vi "FaulhaberV3-Ascii_V1.vi"() -> (1 "searchnames":string[](array[string]), 2 "ID":u32[](array[numeric]), 3 "Faulhaber Objects":T3(array[cluster]))   [LabVIEW 2011] (continued)
Omapping=\"no\" objFlags=\"00020003\" />\n\t\t\t\t\t\t<CANopenSubObject subIndex=\"02\" name=\"Call stack level 1\" objectType=\"7\" dataType=\"0006\" accessType=\"ro\" defaultValue=\"0x0\" PDOmapping=\"no\" objFlags=\"00020003\" />\n\t\t\t\t\t\t<CANopenSubObject subIndex=\"03\" name=\"Call stack level 2\" objectType=\"7\" dataType=\"0006\" accessType=\"ro\" defaultValue=\"0x0\" PDOmapping=\"no\" objFlags=\"00020003\" />\n\t\t\t\t\t\t<CANopenSubObject subIndex=\"04\" name=\"Call stack level 3\" objectType=\"7\" dataType=\"0006\" accessType=\"ro\" defaultValue=\"0x0\" PDOmapping=\"no\" objFlags=\"00020003\" />\n\t\t\t\t\t\t<CANopenSubObject subIndex=\"05\" name=\"Call stack level 4\" objectType=\"7\" dataType=\"0006\" accessType=\"ro\" defaultValue=\"0x0\" PDOmapping=\"no\" objFlags=\"00020003\" />\n\t\t\t\t\t\t<CANopenSubObject subIndex=\"06\" name=\"Call stack level 5\" objectType=\"7\" dataType=\"0006\" accessType=\"ro\" defaultValue=\"0x0\" PDOmapping=\"no\" objFlags=\"00020003\" />\n\t\t\t\t\t\t<CANopenSubObject subIndex=\"07\" name=\"Call stack level 6\" objectType=\"7\" dataType=\"0006\" accessType=\"ro\" defaultValue=\"0x0\" PDOmapping=\"no\" objFlags=\"00020003\" />\n\t\t\t\t\t\t<CANopenSubObject subIndex=\"08\" name=\"Call stack level 7\" objectType=\"7\" dataType=\"0006\" accessType=\"ro\" defaultValue=\"0x0\" PDOmapping=\"no\" objFlags=\"00020003\" />\n\t\t\t\t\t\t<CANopenSubObject subIndex=\"09\" name=\"Call stack level 8\" objectType=\"7\" dataType=\"0006\" accessType=\"ro\" defaultValue=\"0x0\" PDOmapping=\"no\" objFlags=\"00020003\" />\n\t\t\t\t\t\t<CANopenSubObject subIndex=\"0A\" name=\"Call stack level 9\" objectType=\"7\" dataType=\"0006\" accessType=\"ro\" defaultValue=\"0x0\" PDOmapping=\"no\" objFlags=\"00020003\" />\n\t\t\t\t\t\t<CANopenSubObject subIndex=\"0B\" name=\"Call stack level 10\" objectType=\"7\" dataType=\"0006\" accessType=\"ro\" defaultValue=\"0x0\" PDOmapping=\"no\" objFlags=\"00020003\" />\n\t\t\t\t\t\t<CANopenSubObject subIndex=\"0C\" name=\"Call stack level 11\" objectType=\"7\" dataType=\"0006\" accessType=\"ro\" defaultValue=\"0x0\" PDOmapping=\"no\" objFlags=\"00020003\" />\n\t\t\t\t\t\t<CANopenSubObject subIndex=\"0D\" name=\"Call stack level 12\" objectType=\"7\" dataType=\"0006\" accessType=\"ro\" defaultValue=\"0x0\" PDOmapping=\"no\" objFlags=\"00020003\" />\n\t\t\t\t\t\t<CANopenSubObject subIndex=\"0E\" name=\"Call stack level 13\" objectType=\"7\" dataType=\"0006\" accessType=\"ro\" defaultValue=\"0x0\" PDOmapping=\"no\" objFlags=\"00020003\" />\n\t\t\t\t\t\t<CANopenSubObject subIndex=\"0F\" name=\"Call stack level 14\" objectType=\"7\" dataType=\"0006\" accessType=\"ro\" defaultValue=\"0x0\" PDOmapping=\"no\" objFlags=\"00020003\" />\n\t\t\t\t\t</CANopenObject>\n\t\t\t\t\t<CANopenObject index=\"300F\" name=\"Variable access key\" objectType=\"7\" dataType=\"0007\" lowLimit=\"0\" highLimit=\"4294967295\" accessType=\"wo\" defaultValue=\"0\" PDOmapping=\"TPDO\" objFlags=\"00020000\" />\n\t\t\t\t\t<CANopenObject index=\"3010\" name=\"Program constants\" objectType=\"9\" subNumber=\"17\">\n\t\t\t\t\t\t<CANopenSubObject subIndex=\"00\" name=\"Number of entries\" objectType=\"7\" dataType=\"0005\" accessType=\"ro\" defaultValue=\"16\" PDOmapping=\"no\" />\n\t\t\t\t\t\t<CANopenSubObject subIndex=\"01\" name=\"Program constant 0\" objectType=\"7\" dataType=\"0004\" lowLimit=\"-2147483648\" highLimit=\"2147483647\" accessType=\"rw\" defaultValue=\"0\" PDOmapping=\"optional\" />\n\t\t\t\t\t\t<CANopenSubObject subIndex=\"02\" name=\"Program constant 1\" objectType=\"7\" dataType=\"0004\" lowLimit=\"-2147483648\" highLimit=\"2147483647\" accessType=\"rw\" defaultValue=\"0\" PDOmapping=\"optional\" />\n\t\t\t\t\t\t<CANopenSubObject subIndex=\"03\" name=\"Program constant 2\" objectType=\"7\" dataType=\"0004\" lowLimit=\"-2147483648\" highLimit=\"2147483647\" accessType=\"rw\" defaultValue=\"0\" PDOmapping=\"optional\" />\n\t\t\t\t\t\t<CANopenSubObject subIndex=\"04\" name=\"Program constant 3\" objectType=\"7\" dataType=\"0004\" lowLimit=\"-2147483648\" highLimit=\"2147483647\" accessType=\"rw\" defaultValue=\"0\" PDOmapping=\"optional\" />\n\t\t\t\t\t\t<CANopenSubObject subIndex=\"05\" name=\"Program constant 4\" objectType=\"7\" dataType=\"0004\" lowLimit=\"-2147483648\" highLimit=\"2147483647\" accessType=\"rw\" defaultValue=\"0\" PDOmapping=\"optional\" />\n\t\t\t\t\t\t<CANopenSubObject subIndex=\"06\" name=\"Program constant 5\" objectType=\"7\" dataType=\"0004\" lowLimit=\"-2147483648\" highLimit=\"2147483647\" accessType=\"rw\" defaultValue=\"0\" PDOmapping=\"optional\" />\n\t\t\t\t\t\t<CANopenSubObject subIndex=\"07\" name=\"Program constant 6\" objectType=\"7\" dataType=\"0004\" lowLimit=\"-2147483648\" highLimit=\"2147483647\" accessType=\"rw\" defaultValue=\"0\" PDOmapping=\"optional\" />\n\t\t\t\t\t\t<CANopenSubObject subIndex=\"08\" name=\"Program constant 7\" objectType=\"7\" dataType=\"0004\" lowLimit=\"-2147483648\" highLimit=\"2147483647\" accessType=\"rw\" defaultValue=\"0\" PDOmapping=\"optional\" />\n\t\t\t\t\t\t<CANopenSubObject subIndex=\"09\" name=\"Program constant 8\" objectType=\"7\" dataType=\"0004\" lowLimit=\"-2147483648\" highLimit=\"2147483647\" accessType=\"rw\" defaultValue=\"0\" PDOmapping=\"optional\" />\n\t\t\t\t\t\t<CANopenSubObject subIndex=\"0A\" name=\"Program constant 9\" objectType=\"7\" dataType=\"0004\" lowLimit=\"-2147483648\" highLimit=\"2147483647\" accessType=\"rw\" defaultValue=\"0\" PDOmapping=\"optional\" />\n\t\t\t\t\t\t<CANopenSubObject subIndex=\"0B\" name=\"Program constant 10\" objectType=\"7\" dataType=\"0004\" lowLimit=\"-2147483648\" highLimit=\"2147483647\" accessType=\"rw\" defaultValue=\"0\" PDOmapping=\"optional\" />\n\t\t\t\t\t\t<CANopenSubObject subIndex=\"0C\" name=\"Program constant 11\" objectType=\"7\" dataType=\"0004\" lowLimit=\"-2147483648\" highLimit=\"2147483647\" accessType=\"rw\" defaultValue=\"0\" PDOmapping=\"optional\" />\n\t\t\t\t\t\t<CANopenSubObject subIndex=\"0D\" name=\"Program constant 12\" objectType=\"7\" dataType=\"0004\" lowLimit=\"-2147483648\" highLimit=\"2147483647\" accessType=\"rw\" defaultValue=\"0\" PDOmapping=\"optional\" />\n\t\t\t\t\t\t<CANopenSubObject subIndex=\"0E\" name=\"Program constant 13\" objectType=\"7\" dataType=\"0004\" lowLimit=\"-2147483648\" highLimit=\"2147483647\" accessType=\"rw\" defaultValue=\"0\" PDOmapping=\"optional\" />\n\t\t\t\t\t\t<CANopenSubObject subIndex=\"0F\" name=\"Program constant 14\" objectType=\"7\" dataType=\"0004\" lowLimit=\"-2147483648\" highLimit=\"2147483647\" accessType=\"rw\" defaultValue=\"0\" PDOmapping=\"optional\" />\n\t\t\t\t\t\t<CANopenSubObject subIndex=\"10\" name=\"Program constant 15\" objectType=\"7\" dataType=\"0004\" lowLimit=\"-2147483648\" highLimit=\"2147483647\" accessType=\"rw\" defaultValue=\"0\" PDOmapping=\"optional\" />\n\t\t\t\t\t</CANopenObject>\n\t\t\t\t\t<CANopenObject index=\"6007\" name=\"Abort connection option code\" objectType=\"7\" dataType=\"0003\" PDOmapping=\"RPDO\" objFlags=\"00020000\" uniqueIDRef=\"UID_PARAM_6007\" />\n\t\t\t\t\t<CANopenObject index=\"6040\" name=\"Controlword\" objectType=\"7\" dataType=\"0006\" lowLimit=\"0\" highLimit=\"65535\" accessType=\"rw\" defaultValue=\"0x0\" PDOmapping=\"RPDO\" objFlags=\"0001\" />\n\t\t\t\t\t<CANopenObject index=\"6041\" name=\"Statusword\" objectType=\"7\" dataType=\"0006\" lowLimit=\"0x0\" accessType=\"ro\" PDOmapping=\"TPDO\" />\n\t\t\t\t\t<CANopenObject index=\"605A\" name=\"Quick-Stop option code\" objectType=\"7\" dataType=\"0003\" PDOmapping=\"RPDO\" objFlags=\"00020000\" uniqueIDRef=\"UID_PARAM_605A\" />\n\t\t\t\t\t<CANopenObject index=\"605B\" name=\"Shutdown option code\" objectType=\"7\" dataType=\"0003\" PDOmapping=\"RPDO\" objFlags=\"00020000\" uniqueIDRef=\"UID_PARAM_605B\" />\n\t\t\t\t\t<CANopenObject index=\"605C\" name=\"Disable operation option code\" objectType=\"7\" dataType=\"0003\" PDOmapping=\"RPDO\" objFlags=\"00020000\" uniqueIDRef=\"UID_PARAM_605C\" />\n\t\t\t\t\t<CANopenObject index=\"605D\" name=\"Halt option code\" objectType=\"7\" dataType=\"0003\" PDOmapping=\"RPDO\" objFlags=\"00020000\" uniqueIDRef=\"UID_PARAM_605D\" />\n\t\t\t\t\t<CANopenObject index=\"605E\" name=\"Fault reaction option code\" objectType=\"7\" dataType=\"0003\" PDOmapping=\"RPDO\" objFlags=\"00020000\" uniqueIDRef=\"UID_PARAM_605E\" />\n\t\t\t\t\t<CANopenObject index=\"6060\" name=\"Modes of operation\" objectType=\"7\" dataType=\"0002\" PDOmapping=\"RPDO\" objFlags=\"00020000\" uniqueIDRef=\"UID_PARAM_6060\" />\n\t\t\t\t\t<CANopenObject index=\"6061\" name=\"Modes of operation display\" objectType=\"7\" dataType=\"0002\" accessType=\"ro\" PDOmapping=\"TPDO\" objFlags=\"00020000\" />\n\t\t\t\t\t<CANopenObject index=\"6062\" name=\"Position demand value\" objectType=\"7\" dataType=\"0004\" accessType=\"ro\" PDOmapping=\"TPDO\" />\n\t\t\t\t\t<CANopenObject index=\"6063\" name=\"Position actual internal value\" objectType=\"7\" dataType=\"0004\" accessType=\"ro\" PDOmapping=\"TPDO\" />\n\t\t\t\t\t<CANopenObject index=\"6064\" name=\"Position actual value\" objectType=\"7\" dataType=\"0004\" accessType=\"ro\" PDOmapping=\"TPDO\" />\n\t\t\t\t\t<CANopenObject index=\"6065\" name=\"Following error window\" objectType=\"7\" dataType=\"0007\" lowLimit=\"0\" highLimit=\"4294967295\" accessType=\"rw\" PDOmapping=\"RPDO\" objFlags=\"00020000\" />\n\t\t\t\t\t<CANopenObject index=\"6066\" name=\"Following error time out\" objectType=\"7\" dataType=\"0006\" lowLimit=\"1\" highLimit=\"65535\" accessType=\"rw\" PDOmapping=\"RPDO\" objFlags=\"00020000\" />\n\t\t\t\t\t<CANopenObject index=\"6067\" name=\"Position window\" objectType=\"7\" dataType=\"0007\" lowLimit=\"0\" highLimit=\"4294967295\" accessType=\"rw\" PDOmapping=\"RPDO\" objFlags=\"00020000\" />\n\t\t\t\t\t<CANopenObject index=\"6068\" name=\"Position window time\" objectType=\"7\" dataType=\"0006\" lowLimit=\"1\" highLimit=\"65535\" accessType=\"rw\" PDOmapping=\"RPDO\" objFlags=\"00020000\" />\n\t\t\t\t\t<CANopenObject index=\"606B\" name=\"Velocity demand value\" objectType=\"7\" dataType=\"0004\" accessType=\"ro\" PDOmapping=\"TPDO\" />\n\t\t\t\t\t<CANopenObject index=\"606C\" name=\"Velocity actual value\" objectType=\"7\" dataType=\"0004\" accessType=\"ro\" PDOmapping=\"TPDO\" />\n\t\t\t\t\t<CANopenObject index=\"606D\" name=\"Velocity window\" objectType=\"7\" dataType=\"0006\" lowLimit=\"0\" highLimit=\"65535\" accessType=\"rw\" PDOmapping=\"RPDO\" objFlags=\"00020000\" />\n\t\t\t\t\t<CANopenObject index=\"606E\" name=\"Velocity window time\" objectType=\"7\" dataType=\"0006\" lowLimit=\"1\" highLimit=\"65535\" accessType=\"rw\" PDOmapping=\"RPDO\" objFlags=\"00020000\" />\n\t\t\t\t\t<CANopenObject index=\"606F\" name=\"Velocity threshold\" objectType=\"7\" dataType=\"0006\" lowLimit=\"0\" highLimit=\"65535\" accessType=\"rw\" PDOmapping=\"RPDO\" objFlags=\"00020000\" />\n\t\t\t\t\t<CANopenObject index=\"6070\" name=\"Velocity threshold time\" objectType=\"7\" dataType=\"0006\" lowLimit=\"1\" highLimit=\"65535\" accessType=\"rw\" PDOmapping=\"RPDO\" objFlags=\"00020000\" />\n\t\t\t\t\t<CANopenObject index=\"6071\" name=\"Target torque\" objectType=\"7\" dataType=\"0003\" lowLimit=\"-32768\" highLimit=\"32767\" accessType=\"rw\" defaultValue=\"0\" PDOmapping=\"RPDO\" />\n\t\t\t\t\t<CANopenObject index=\"6072\" name=\"Max torque\" objectType=\"7\" dataType=\"0006\" accessType=\"ro\" PDOmapping=\"TPDO\" />\n\t\t\t\t\t<CANopenObject index=\"6074\" name=\"Torque demand\" objectType=\"7\" dataType=\"0003\" accessType=\"ro\" PDOmapping=\"TPDO\" />\n\t\t\t\t\t<CANopenObject index=\"6077\" name=\"Torque actual value\" objectType=\"7\" dataType=\"0003\" accessType=\"ro\" PDOmapping=\"TPDO\" />\n\t\t\t\t\t<CANopenObject index=\"6078\" name=\"Current actual value\" objectType=\"7\" dataType=\"0003\" accessType=\"ro\" PDOmapping=\"TPDO\" />\n\t\t\t\t\t<CANopenObject index=\"607A\" name=\"Target position\" objectType=\"7\" dataType=\"0004\" lowLimit=\"-2147483648\" highLimit=\"2147483647\" accessType=\"rw\" defaultValue=\"0\" PDOmapping=\"RPDO\" />\n\t\t\t\t\t<CANopenObject index=\"607B\" name=\"Position range limit\" objectType=\"8\" subNumber=\"3\">\n\t\t\t\t\t\t<CANopenSubObject subIndex=\"00\" name=\"Number of entries\" objectType=\"7\" dataType=\"0005\" accessType=\"ro\" defaultValue=\"2\" PDOmapping=\"no\" />\n\t\t\t\t\t\t<CANopenSubObject subIndex=\"01\" name=\"Min position range limit\" objectType=\"7\" dataType=\"0004\" lowLimit=\"-2147483648\" highLimit=\"2147483647\" accessType=\"rw\" defaultValue=\"-2147483648\" PDOmapping=\"RPDO\" objFlags=\"00020000\" />\n\t\t\t\t\t\t<CANopenSubObject subIndex=\"02\" name=\"Max position range limit\" objectType=\"7\" dataType=\"0004\" lowLimit=\"-2147483648\" highLimit=\"2147483647\" accessType=\"rw\" defaultValue=\"2147483647\" PDOmapping=\"RPDO\" objFlags=\"00020000\" />\n\t\t\t\t\t</CANopenObject>\n\t\t\t\t\t<CANopenObject index=\"607C\" name=\"Home offset\" objectType=\"7\" dataType=\"0004\" lowLimit=\"-2147483648\" highLimit=\"2147483647\" accessType=\"rw\" defaultValue=\"0\" PDOmapping=\"RPDO\" objFlags=\"00020000\" />\n\t\t\t\t\t<CANopenObject index=\"607D\" name=\"Software position limit\" objectType=\"8\" subNumber=\"3\">\n\t\t\t\t\t\t<CANopenSubObject subIndex=\"00\" name=\"Number of entries\" objectType=\"7\" dataType=\"0005\" accessType=\"ro\" defaultValue=\"2\" PDOmapping=\"no\" />\n\t\t\t\t\t\t<CANopenSubObject subIndex=\"01\" name=\"Min position limit\" objectType=\"7\" dataType=\"0004\" lowLimit=\"-2147483648\" highLimit=\"2147483647\" accessType=\"rw\" defaultValue=\"-2147483648\" PDOmapping=\"RPDO\" objFlags=\"00020000\" />\n\t\t\t\t\t\t<CANopenSubObject subIndex=\"02\" name=\"Max position limit\" objectType=\"7\" dataType=\"0004\" lowLimit=\"-2147483648\" highLimit=\"2147483647\" accessType=\"rw\" defaultValue=\"2147483647\" PDOmapping=\"RPDO\" objFlags=\"00020000\" />\n\t\t\t\t\t</CANopenObject>\n\t\t\t\t\t<CANopenObject index=\"607E\" name=\"Polarity\" objectType=\"7\" dataType=\"0005\" PDOmapping=\"RPDO\" objFlags=\"00020000\" uniqueIDRef=\"UID_PARAM_607E\" />\n\t\t\t\t\t<CANopenObject index=\"6080\" name=\"Max motor speed \" objectType=\"7\" dataType=\"0007\" lowLimit=\"1\" highLimit=\"4294967295\" accessType=\"rw\" defaultValue=\"32767\" PDOmapping=\"RPDO\" />\n\t\t\t\t\t<CANopenObject index=\"6081\" name=\"Profile velocity\" objectType=\"7\" dataType=\"0007\" lowLimit=\"1\" highLimit=\"4294967295\" accessType=\"rw\" defaultValue=\"32767\" PDOmapping=\"RPDO\" />\n\t\t\t\t\t<CANopenObject index=\"6083\" name=\"Profile acceleration\" objectType=\"7\" dataType=\"0007\" lowLimit=\"1\" highLimit=\"32767\" accessType=\"rw\" defaultValue=\"30000\" PDOmapping=\"RPDO\" />\n\t\t\t\t\t<CANopenObject index=\"6084\" name=\"Profile deceleration\" objectType=\"7\" dataType=\"0007\" lowLimit=\"1\" highLimit=\"32767\" accessType=\"rw\" defaultValue=\"30000\" PDOmapping=\"RPDO\" />\n\t\t\t\t\t<CANopenObject index=\"6085\" name=\"Quick stop deceleration\" objectType=\"7\" dataType=\"0007\" lowLimit=\"10\" highLimit=\"32767\" accessType=\"rw\" defaultValue=\"30000\" PDOmapping=\"RPDO\" />\n\t\t\t\t\t<CANopenObject index=\"6086\" name=\"Motion profile type\" objectType=\"7\" dataType=\"0003\" PDOmapping=\"RPDO\" objFlags=\"00020000\" uniqueIDRef=\"UID_PARAM_6086\" />\n\t\t\t\t\t<CANopenObject index=\"608F\" name=\"Position encoder resolution\" objectType=\"8\" subNumber=\"3\">\n\t\t\t\t\t\t<CANopenSubObject subIndex=\"00\" name=\"Number of entries\" objectType=\"7\" dataType=\"0005\" accessType=\"ro\" defaultValue=\"2\" PDOmapping=\"no\" />\n\t\t\t\t\t\t<CANopenSubObject subIndex=\"01\" name=\"Encoder increments\" objectType=\"7\" dataType=\"0007\" accessType=\"ro\" PDOmapping=\"no\" objFlags=\"00020000\" />\n\t\t\t\t\t\t<CANopenSubObject subIndex=\"02\" name=\"Motor revolutions\" objectType=\"7\" dataType=\"0007\" accessType=\"ro\" PDOmapping=\"no\" objFlags=\"00020000\" />\n\t\t\t\t\t</CANopenObject>\n\t\t\t\t\t<CANopenObject index=\"6090\" name=\"Velocity encoder resolution\" objectType=\"8\" subNumber=\"3\">\n\t\t\t\t\t\t<CANopenSubObject subIndex=\"00\" name=\"Number of entries\" objectType=\"7\" dataType=\"0005\" accessType=\"ro\" defaultValue=\"2\" PDOmapping=\"no\" />\n\t\t\t\t\t\t<CANopenSubObject subIndex=\"01\" name=\"Encoder increments\" objectType=\"7\" dataType=\"0007\" accessType=\"ro\" PDOmapping=\"no\" objFlags=\"00020000\" />\n\t\t\t\t\t\t<CANopenSubObject subIndex=\"02\" name=\"Motor revolutions\" objectType=\"7\" dataType=\"0007\" accessType=\"ro\" PDOmapping=\"no\" objFlags=\"00020000\" />\n\t\t\t\t\t</CANopenObject>\n\t\t\t\t\t<CANopenObject index=\"6091\" name=\"Gear ratio\" objectType=\"8\" subNumber=\"3\">\n\t\t\t\t\t\t<CANopenSubObject subIndex=\"00\" name=\"Number of entries\" objectType=\"7\" dataType=\"0005\" accessType=\"ro\" defaultValue=\"2\" PDOmapping=\"no\" />\n\t\t\t\t\t\t<CANopenSubObject subIndex=\"01\" name=\"Motor shaft revolutions\" objectType=\"7\" dataType=\"0007\" lowLimit=\"1\" highLimit=\"4294967295\" accessType=\"rw\" defaultValue=\"1\" PDOmapping=\"RPDO\" objFlags=\"00020000\" />\n\t\t\t\t\t\t<CANopenSubObject subIndex=\"02\" name=\"Driving shaft revolutions\" objectType=\"7\" dataType=\"0007\" lowLimit=\"1\" highLimit=\"4294967295\" accessType=\"rw\" defaultValue=\"1\" PDOmapping=\"RPDO\" objFlags=\"00020000\" />\n\t\t\t\t\t</CANopenObject>\n\t\t\t\t\t<CANopenObject index=\"6092\" name=\"Feed constant\" objectType=\"8\" subNumber=\"3\">\n\t\t\t\t\t\t<CANopenSubObject subIndex=\"00\" name=\"Number of entries\" objectType=\"7\" dataType=\"0005\" accessType=\"ro\" defaultValue=\"2\" PDOmapping=\"no\" />\n\t\t\t\t\t\t<CANopenSubObject subIndex=\"01\" name=\"Feed\" objectType=\"7\" dataType=\"0007\" lowLimit=\"1\" highLimit=\"4294967295\" accessType=\"rw\" defaultValue=\"4096\" PDOmapping=\"RPDO\" objFlags=\"00020000\" />\n\t\t\t\t\t\t<CANopenSubObject subIndex=\"02\" name=\"Shaft revolutions\" objectType=\"7\" dataType=\"0007\" lowLimit=\"1\" highLimit=\"4294967295\" accessType=\"rw\" defaultValue=\"1\" PDOmapping=\"RPDO\" objFlags=\"00020000\" />\n\t\t\t\t\t</CANopenObject>\n\t\t\t\t\t<CANopenObject index=\"6096\" name=\"Velocity factor\" objectType=\"8\" subNumber=\"3\">\n\t\t\t\t\t\t<CANopenSubObject subIndex=\"00\" name=\"Number of entries\" objectType=\"7\" dataType=\"0005\" accessType=\"ro\" defaultValue=\"2\" PDOmapping=\"no\" />\n\t\t\t\t\t\t<CANopenSubObject subIndex=\"01\" name=\"Numerator\" objectType=\"7\" dataType=\"0007\" lowLimit=\"1\" highLimit=\"4294967295\" accessType=\"rw\" defaultValue=\"1\" PDOmapping=\"RPDO\" objFlags=\"00020000\" />\n\t\t\t\t\t\t<CANopenSubObject subIndex=\"02\" name=\"Divisor\" objectType=\"7\" dataType=\"0007\" lowLimit=\"1\" highLimit=\"4294967295\" accessType=\"rw\" defaultValue=\"4096\" PDOmapping=\"RPDO\" objFlags=\"00020000\" />\n\t\t\t\t\t</CANopenObject>\n\t\t\t\t\t<CANopenObject index=\"6098\" name=\"Homing method\" objectType=\"7\" dataType=\"0002\" lowLimit=\"-4\" highLimit=\"37\" accessType=\"rw\" defaultValue=\"0\" PDOmapping=\"RPDO\" objFlags=\"00020000\" />\n\t\t\t\t\t<CANopenObject index=\"6099\" name=\"Homing speeds\" objectType=\"8\" subNumber=\"3\">\n\t\t\t\t\t\t<CANopenSubObject subIndex=\"00\" name=\"Number of entries\" objectType=\"7\" dataType=\"0005\" accessType=\"ro\" defaultValue=\"2\" PDOmapping=\"no\" />\n\t\t\t\t\t\t<CANopenSubObject subIndex=\"01\" name=\"Switch seek velocity\" objectType=\"7\" dataType=\"0007\" lowLimit=\"0\" highLimit=\"4294967295\" accessType=\"rw\" defaultValue=\"400\" PDOmapping=\"RPDO\" objFlags=\"00020000\" />\n\t\t\t\t\t\t<CANopenSubObject subIndex=\"02\" name=\"Homing speed\" objectType=\"7\" dataType=\"0007\" lowLimit=\"0\" highLimit=\"4294967295\" accessType=\"rw\" defaultValue=\"400\" PDOmapping=\"RPDO\" objFlags=\"00020000\" />\n\t\t\t\t\t</CANopenObject>\n\t\t\t\t\t<CANopenObject index=\"609A\" name=\"Homing acceleration\" objectType=\"7\" dataType=\"0007\" lowLimit=\"0\" highLimit=\"4294967295\" accessType=\"rw\" defaultValue=\"50\" PDOmapping=\"RPDO\" objFlags=\"00020000\" />\n\t\t\t\t\t<CANopenObject index=\"60B0\" name=\"Position offset\" objectType=\"7\" dataType=\"0004\" lowLimit=\"-2147483648\" highLimit=\"2147483647\" accessType=\"rw\" defaultValue=\"0\" PDOmapping=\"RPDO\" />\n\t\t\t\t\t<CANopenObject index=\"60B1\" name=\"Velocity offset\" objectType=\"7\" dataType=\"0004\" lowLimit=\"-2147483648\" highLimit=\"2147483647\" accessType=\"rw\" defaultValue=\"0\" PDOmapping=\"RPDO\" />\n\t\t\t\t\t<CANopenObject index=\"60B2\" name=\"Torque offset\" objectType=\"7\" dataType=\"0003\" lowLimit=\"-32768\" highLimit=\"32767\" accessType=\"rw\" defaultValue=\"0\" PDOmapping=\"RPDO\" />\n\t\t\t\t\t<CANopenObject index=\"60B8\" name=\"Touch probe function\" objectType=\"7\" dataType=\"0006\" accessType=\"rw\" defaultValue=\"0\" PDOmapping=\"RPDO\" />\n\t\t\t\t\t<CANopenObject index=\"60B9\" name=\"Touch probe status\" objectType=\"7\" dataType=\"0006\" accessType=\"ro\" defaultValue=\"0x0000\" PDOmapping=\"TPDO\" />\n\t\t\t\t\t<CANopenObject index=\"60BA\" name=\"Touch probe 1 positive edge\" objectType=\"7\" dataType=\"0004\" accessType=\"ro\" defaultValue=\"0x0000\" PDOmapping=\"TPDO\" />\n\t\t\t\t\t<CANopenObject index=\"60BB\" name=\"Touch probe 1 negative edge\" objectType=\"7\" dataType=\"0004\" accessType=\"ro\" PDOmapping=\"TPDO\" />\n\t\t\t\t\t<CANopenObject index=\"60BC\" name=\"Touch probe 2 positive edge\" objectType=\"7\" dataType=\"0004\" accessType=\"ro\" PDOmapping=\"TPDO\" />\n\t\t\t\t\t<CANopenObject index=\"60BD\" name=\"Touch probe 2 negative edge\" objectType=\"7\" dataType=\"0004\" accessType=\"ro\" PDOmapping=\"TPDO\" />\n\t\t\t\t\t<CANopenObject index=\"60C5\" name=\"Max acceleration\" objectType=\"7\" dataType=\"0007\" lowLimit=\"10\" highLimit=\"32767\" accessType=\"rw\" defaultValue=\"30000\" PDOmapping=\"RPDO\" objFlags=\"00020000\" />\n\t\t\t\t\t<CANopenObject index=\"60C6\" name=\"Max deceleration\" objectType=\"7\" dataType=\"0007\" lowLimit=\"10\" highLimit=\"32767\" accessType=\"rw\" defaultValue=\"30000\" PDOmapping=\"RPDO\" objFlags=\"00020000\" />\n\t\t\t\t\t<CANopenObject index=\"60D5\" name=\"Touch probe 1 positive edge counter\" objectType=\"7\" dataType=\"0006\" accessType=\"ro\" PDOmapping=\"TPDO\" />\n\t\t\t\t\t<CANopenObject index=\"60D6\" name=\"Touch probe 1 negative edge counter\" objectType=\"7\" dataType=\"0006\" accessType=\"ro\" PDOmapping=\"TPDO\" />\n\t\t\t\t\t<CANopenObject index=\"60D7\" name=\"Touch probe 2 positive edge counter\" objectType=\"7\" dataType=\"0006\" accessType=\"ro\" PDOmapping=\"TPDO\" />\n\t\t\t\t\t<CANopenObject index=\"60D8\" name=\"Touch probe 2 negative edge counter\" objectType=\"7\" dataType=\"0006\" accessType=\"ro\" PDOmapping=\"TPDO\" />\n\t\t\t\t\t<CANopenObject index=\"60E0\" name=\"Positive torque limit value\" objectType=\"7\" dataType=\"0006\" lowLimit=\"0\" highLimit=\"6000\" accessType=\"rw\" defaultValue=\"2000\" PDOmapping=\"RPDO\" />\n\t\t\t\t\t<CANopenObject index=\"60E1\" name=\"Negative torque limit value\" objectType=\"7\" dataType=\"0006\" lowLimit=\"0\" highLimit=\"6000\" accessType=\"rw\" defaultValue=\"2000\" PDOmapping=\"RPDO\" />\n\t\t\t\t\t<CANopenObject index=\"60F2\" name=\"Position option code\" objectType=\"7\" dataType=\"0006\" PDOmapping=\"RPDO\" objFlags=\"00020000\" uniqueIDRef=\"UID_PARAM_60F2\" />\n\t\t\t\t\t<CANopenObject index=\"60F4\" name=\"Following error actual value\" objectType=\"7\" dataType=\"0004\" accessType=\"ro\" PDOmapping=\"TPDO\" />\n\t\t\t\t\t<CANopenObject index=\"60FD\" name=\"Digital Inputs\" objectType=\"7\" dataType=\"0007\" accessType=\"ro\" PDOmapping=\"TPDO\" />\n\t\t\t\t\t<CANopenObject index=\"60FF\" name=\"Target velocity\" objectType=\"7\" dataType=\"0004\" lowLimit=\"-2147483648\" highLimit=\"2147483647\" accessType=\"rw\" defaultValue=\"0\" PDOmapping=\"RPDO\" />\n\t\t\t\t\t<CANopenObject index=\"6403\" name=\"Motor catalogue number\" objectType=\"7\" dataType=\"0009\" accessType=\"ro\" PDOmapping=\"no\" objFlags=\"00020000\" />\n\t\t\t\t\t<CANopenObject index=\"6502\" name=\"Supported drive modes\" objectType=\"7\" dataType=\"0007\" accessType=\"ro\" PDOmapping=\"TPDO\" objFlags=\"00020000\" />\n\t\t\t\t\t<CANopenObject index=\"6503\" name=\"Drive catalogue number\" objectType=\"7\" dataType=\"0009\" accessType=\"const\" defaultValue=\"0\" PDOmapping=\"no\" objFlags=\"00020000\" />\n\t\t\t\t</CANopenObjectList>\n\t\t\t\t<dummyUsage>\n\t\t\t\t\t<dummy entry=\"Dummy0001=0\" />\n\t\t\t\t\t<dummy entry=\"Dummy0002=0\" />\n\t\t\t\t\t<dummy entry=\"Dummy0003=0\" />\n\t\t\t\t\t<dummy entry=\"Dummy0004=0\" />\n\t\t\t\t\t<dummy entry=\"Dummy0005=0\" />\n\t\t\t\t\t<dummy entry=\"Dummy0006=0\" />\n\t\t\t\t\t<dummy entry=\"Dummy0007=0\" />\n\t\t\t\t</dummyUsage>\n\t\t\t</ApplicationLayers>\n\t\t\t<TransportLayers>\n\t\t\t\t<PhysicalLayer>\n\t\t\t\t\t<baudRate defaultValue=\"250 Kbps\">\n\t\t\t\t\t\t<supportedBaudRate value=\"20 Kbps\" />\n\t\t\t\t\t\t<supportedBaudRate value=\"50 Kbps\" />\n\t\t\t\t\t\t<supportedBaudRate value=\"125 Kbps\" />\n\t\t\t\t\t\t<supportedBaudRate value=\"250 Kbps\" />\n\t\t\t\t\t\t<supportedBaudRate value=\"500 Kbps\" />\n\t\t\t\t\t\t<supportedBaudRate value=\"1000 Kbps\" />\n\t\t\t\t\t</baudRate>\n\t\t\t\t</PhysicalLayer>\n\t\t\t</TransportLayers>\n\t\t\t<NetworkManagement>\n\t\t\t\t<CANopenGeneralFeatures groupMessaging=\"false\" dynamicChannels=\"0\" selfStartingDevice=\"false\" SDORequestingDevice=\"false\" granularity=\"4\" nrOfRxPDO=\"4\" nrOfTxPDO=\"4\" bootUpSlave=\"false\" layerSettingServiceSlave=\"true\" />\n\t\t\t\t<CANopenMasterFeatures bootUpMaster=\"false\" flyingMaster=\"false\" SDOManager=\"false\" configurationManager=\"false\" layerSettingServiceMaster=\"true\" />\n\t\t\t\t<deviceCommissioning nodeID=\"1\" nodeName=\"\" actualBaudRate=\"250\" networkNumber=\"0\" networkName=\"\" CANopenManager=\"false\" />\n\t\t\t</NetworkManagement>\n\t\t</ProfileBody>\n\t</ISO15745Profile>\n</ISO15745ProfileContainer>"
  # "tabs"
  # "objekttype7 Normal\nobjectType=\"8\"  nur header, gibt subindex extra"
  # "datatype\n1 gibt nicht\n2: S8  ,1x da6098 \n3: S16\n4: S32\n5:U16\n6: U16\n7:U32\n8: nie\n9 Strimg?"
  # "min/max/default als string?"
  # "accesstype\nro\nrw"
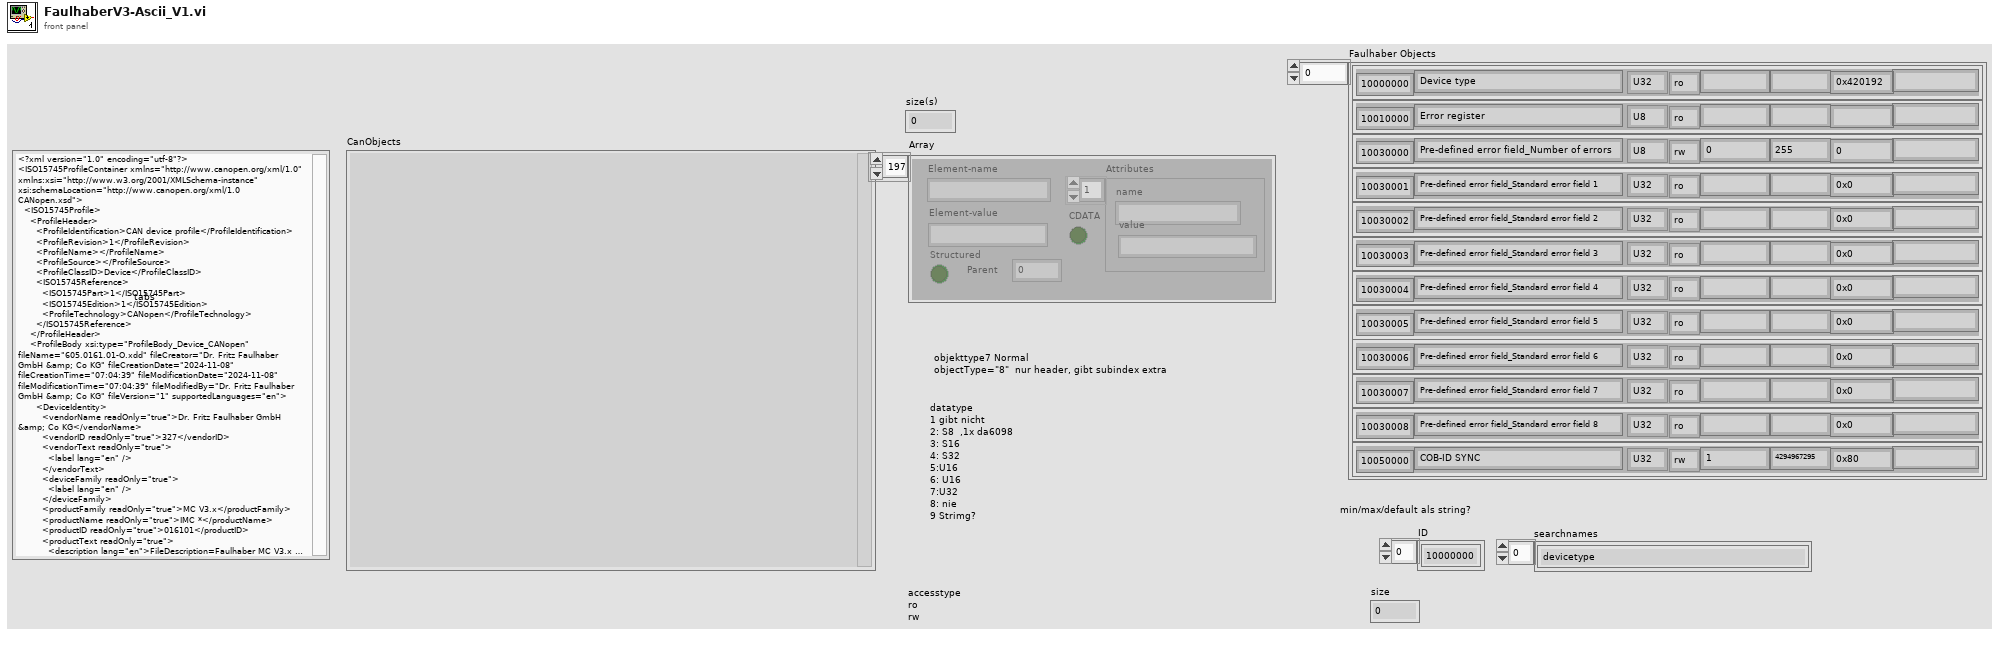
[diagram p1: front panel]
types:
  T1 = typedef "FaulaberType.ctl" = enum8{"unknown", "none", "S8", "S16", "S32", "U8", "U16", "U32", "R", "string"}
  T2 = typedef "FaulhaberAccess.ctl" = enum16{"unknown", "ro", "rw", "wo", "const"}
  T3 = cluster{"ID":u32, "Name":string, "type":T1, "rw":T2, "lowLimit":string, "highLimit":string, "Default":string, "Kommentart":string}[]
  T4 = typedef "MSXML Element.ctl" = cluster{"Element-name":string, "Attributes":T5[], "Element-value":string, "CDATA":bool, "Parent":i32, "Structured":bool}
  T5 = typedef "MSXML attribute.ctl" = cluster{"name":string, "value":string}
  T6 = cluster{"ID":u32, "Name":string, "type":enum8{"unknown", "none", "S8", "S16", "S32", "U8", "U16", "U32", "R", "string"}, "rw":enum16{"unknown", "ro", "rw", "wo", "const"}, "lowLimit":string, "highLimit":string, "Default":string, "Kommentar":string}[]
  T7 = cluster{u32, string, u32, "rw 3":enum16{"unknown", "ro", "rw", "wo", "const"}, "value":string, "value":string, "value":string, string}
  T8 = cluster{"ID":u32, "Name":string, "type":u32, "rw 3":enum16{"unknown", "ro", "rw", "wo", "const"}, "value":string, "value":string, "value":string, "Kommentar":string}[]
  T9 = cluster{"ID":u32, "Name":string, "type":u32, "rw":enum16{"unknown", "ro", "rw", "wo", "const"}, "lowLimit":string, "highLimit":string, "Default":string, "Kommentar":string}
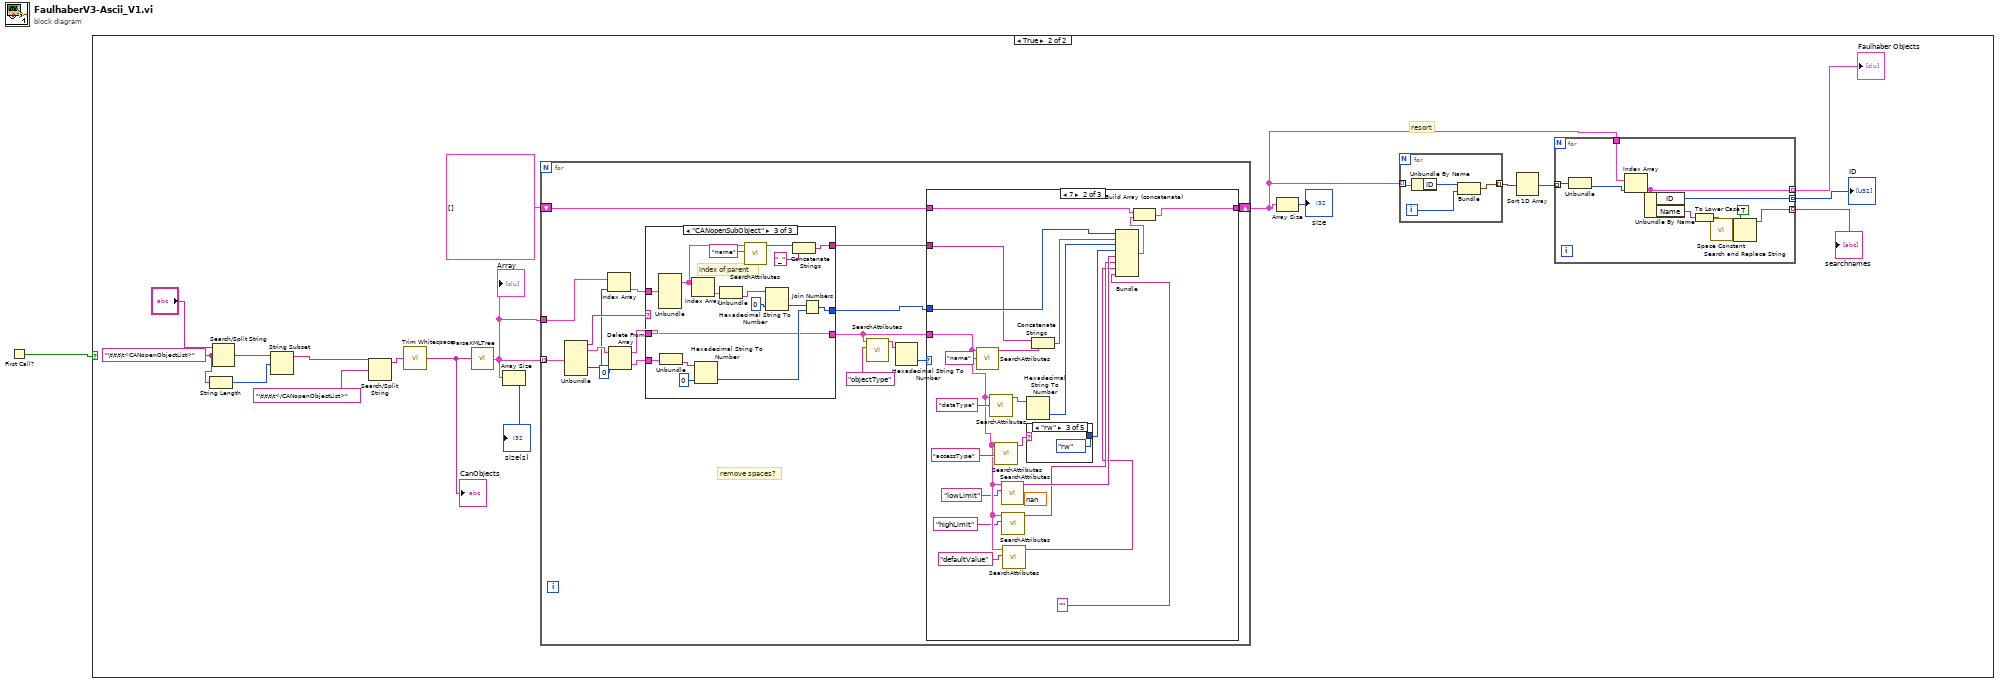
[diagram p0: block diagram]
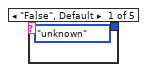
[diagram p4: hidden frame]
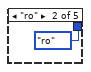
[diagram p5: hidden frame]
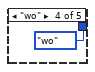
[diagram p6: hidden frame]
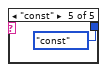
[diagram p7: hidden frame]
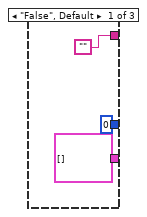
[diagram p9: hidden frame]
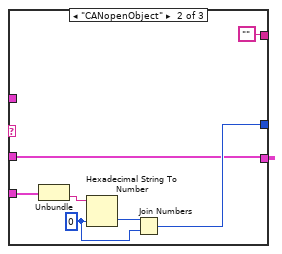
[diagram p10: hidden frame]
diagram:
  n1 = First Call?() -> (First Call?: T/F=w1:bool)
  n2 = case shown="True" w1 {
    frame False {
    }
    frame True {
      w11 = "\t\t\t\t<CANopenObjectList>" ("search string/char (-)")
      # "resort"
      n3 = String Length(string=w11) -> (length=w10:i32)
      n4 = Search/Split String(string="?", search string/char (-)=w11) -> (match + rest of string=w15:string)  [unwired: 1 in, 2 out]
      n5 = String Subset(string=w15, offset (0)=w10) -> (substring=w12:string)  [unwired: 1 in]
      n6 = Search/Split String(string=w12, search string/char (-)="\t\t\t\t</CANopenObjectList>") -> (substring before match=w13:string)  [unwired: 1 in, 2 out]
      n7 = call <vilib>:"Trim Whitespace.vi"("string"=w13) -> ("trimmed string"=w9:string)  [unwired: 1 in]
      "CanObjects" <- w9
      n8 = call "ParseXMLTree.vi"("xml text"=w9) -> ("Array"=w8:T4[])
      "Array" <- w8
      n9 = Array Size(array=w8) -> (size(s)=→"size(s)":i32)
      n10 = for {
        tunnel: w8 -> [w50] mode=indexing
        tunnel: w8 -> [w44]
        shift-right: [w34] -> w3
        shift-left: T6 [] -> [w35]
        # "remove spaces?"
        n11 = Unbundle(w50) -> ("Element-name"=w49:string, "Attributes"=w48:T5[], "Parent"=w45:i32)  [unwired: 3 out]
        n12 = Index Array(array=w44, index=w45) -> (element=w43:T4)
        n13 = Delete From Array(array=w48, index=0) -> (deleted portion=w46:T5, array with subset deleted=w47:T5[])  [unwired: 1 in]
        n14 = case shown="\"CANopenSubObject\"" w49 {
          tunnel: w46 -> [_ w89 w99]
          tunnel: [u32 0 w85 w96] -> w36
          tunnel: w47 -> [_ w84 w95]
          tunnel: [T5[] [] ("Attributes") w84 w95] -> w40
          tunnel: w43 -> [_ _ w105]
          tunnel: ["" "" w92] -> w41
          frame "False", Default {
          }
          frame "CANopenObject" {
            w86 = u16 0 ("default (0 U32)")
            n15 = Unbundle(w89) -> ("value"=w88:string)  [unwired: 1 out]
            n16 = Hexadecimal String To Number(string=w88, default (0uL)=w86) -> (number=w87:u16)  [unwired: 1 in, 1 out]
            n17 = Join Numbers(hi=w87, lo=w86) -> ((hi.lo)=w85:u32)
          }
          frame "CANopenSubObject" {
            # "index of parent"
            n18 = Unbundle(w105) -> ("Attributes"=w94:T5[])  [unwired: 5 out]
            n19 = Unbundle(w99) -> ("value"=w101:string)  [unwired: 1 out]
            n20 = Index Array(array=w94) -> (element=w104:T5)  [unwired: 1 in]
            n21 = Hexadecimal String To Number(string=w101, default (0uL)=u16 0 ("default (0 U32)")) -> (number=w97:u16)  [unwired: 1 in, 1 out]
            n22 = Unbundle(w104) -> ("value"=w102:string)  [unwired: 1 out]
            n23 = call "SearchAttributes.vi"("String"="name", "Attributes"=w94) -> ("value"=w91:string)  [unwired: 8 in, 1 out]
            n24 = Hexadecimal String To Number(string=w102, default (0uL)=u16 0 ("default (0 U32)")) -> (number=w98:u16)  [unwired: 1 in, 1 out]
            n25 = Concatenate Strings(w91, "_" ("string")) -> (w92:string)
            n26 = Join Numbers(hi=w98, lo=w97) -> ((hi.lo)=w96:u32)
          }
        }
        n27 = call "SearchAttributes.vi"("String"="objectType", "Attributes"=w40) -> ("value"=w38:string)  [unwired: 8 in, 1 out]
        n28 = Hexadecimal String To Number(string=w38) -> (number=w37:u32)  [unwired: 2 in, 1 out]
        n29 = case shown="7" w37 {
          tunnel: w41 -> [_ w61 _]
          tunnel: w40 -> [_ w60 _]
          tunnel: w36 -> [_ w64 _]
          tunnel: w35 -> [w51 w65 w79]
          tunnel: [w51 w66 w79] -> w34
          frame 0, Default {
          }
          frame 7 {
            (unwired) nan ("default value 1")
            n30 = call "SearchAttributes.vi"("String"="name", "Attributes"=w60) -> ("value"=w72:string)  [unwired: 8 in, 1 out]
            n31 = call "SearchAttributes.vi"("String"="dataType", "Attributes"=w60) -> ("value"=w70:string)  [unwired: 8 in, 1 out]
            n32 = call "SearchAttributes.vi"("String"="accessType", "Attributes"=w60) -> ("value"=w68:string)  [unwired: 8 in, 1 out]
            n33 = call "SearchAttributes.vi"("String"="lowLimit", "Attributes"=w60) -> ("value"=w55:string)  [unwired: 8 in, 1 out]
            n34 = call "SearchAttributes.vi"("String"="highLimit", "Attributes"=w60) -> ("value"=w54:string)  [unwired: 8 in, 1 out]
            n35 = call "SearchAttributes.vi"("String"="defaultValue", "Attributes"=w60) -> ("value"=w53:string)  [unwired: 8 in, 1 out]
            n36 = Hexadecimal String To Number(string=w70) -> (number=w63:u32)  [unwired: 2 in, 1 out]
            n37 = case shown="\"rw\"" w68 {
              tunnel: [enum16{"unknown", "ro", "rw", "wo", "const"}."unknown" ("rw 3") enum16{"unknown", "ro", "rw", "wo", "const"}."ro" ("rw 3") enum16{"unknown", "ro", "rw", "wo", "const"}."rw" ("rw 3") enum16{"unknown", "ro", "rw", "wo", "const"}."wo" ("rw 3") enum16{"unknown", "ro", "rw", "wo", "const"}."const" ("rw 3")] -> w62
              frame "False", Default {
              }
              frame "ro" {
              }
              frame "rw" {
              }
              frame "wo" {
              }
              frame "const" {
              }
            }
            n38 = Concatenate Strings(w61, w72) -> (w57:string)
            n39 = Bundle(w64, w57, w63, "rw 3"=w62, "value"=w55, "value"=w54, "value"=w53, "") -> (w52:T7)  [unwired: 1 in]
            n40 = Build Array (concatenate)(w65, w52) -> (w66:T8)
          }
          frame 8 {
          }
        }
      }
      n41 = Array Size(array=w3) -> (size(s)=→"size":i32)
      n42 = for {
        tunnel: w3 -> [w33] mode=indexing
        tunnel: [w30] -> w4 mode=indexing
        i -> [w31]
        n43 = Unbundle By Name(w33) -> ("ID"=w32:u32)
        n44 = Bundle("ID"=w32, w31) -> (w30:cluster{"ID":u32, i32})  [unwired: 1 in]
      }
      n45 = Sort 1D Array(array=w4) -> (sorted array=w2:cluster{"ID":u32, i32}[])
      n46 = for {
        tunnel: w3 -> [w28]
        tunnel: w2 -> [w29] mode=indexing
        tunnel: [w26] -> w17 mode=indexing
        tunnel: [w25] -> w19 mode=indexing
        tunnel: [w20] -> w18 mode=indexing
        n47 = Unbundle(w29) -> (w27:i32)  [unwired: 1 out]
        n48 = Index Array(array=w28, index=w27) -> (element=w26:T9)
        n49 = Unbundle By Name(w26) -> ("ID"=w25:u32, "Name"=w21:string)
        n50 = To Lower Case(string=w21) -> (all lower case string=w22:string)
        n51 = call <vilib>:"Space Constant.vi"() -> ("String"=w24:string)
        n52 = Search and Replace String(replace all?=TRUE ("replace all? (F)"), input string=w22, search string=w24) -> (result string=w20:string)  [unwired: 5 in, 3 out]
      }
      "Faulhaber Objects" <- w17
      "ID" <- w19
      "searchnames" <- w18
    }
  }
